vi "Loop_Auto.vi"() -> ()   [LabVIEW 2016, in "TemplateAutonomous.lvlib"]
uses:
  TemplateAutonomous.lvlib
  ENUM_Auto_State.ctl
  ENUM_Auto_Action.ctl
  Globals/Global_STOP.vi
panel:
  out "Input DBL Data":dbl
  out "Output Bool Data":bool
  out "Output DBL Data":dbl
  out "OutputI INT Data":i32
  out "Cycle Time (S)":dbl format="%.3g"
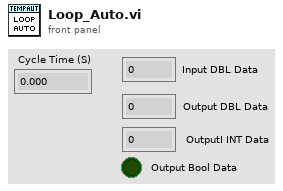
[diagram p1: front panel]
types:
  T1 = typedef "TemplateAutonomous.lvlib/ENUM_Auto_State.ctl" = enum16{"Startup", "Idle", "Auto Step 1", "Auto Step 2", "Shutdown"}
  T2 = typedef "TemplateAutonomous.lvlib/ENUM_Auto_Action.ctl" = enum16{"No Action", "Reset Time", "Reset All", "Action A", "Action B"}
  T3 = cluster{"State":T1, "Previous State":T1, "Current Time":timestamp, "Previous Time":timestamp, "Start Time":timestamp, "Target Time (ms)":u32, "Cycle Time(S)":dbl, "Auto Input DBL":dbl, "Auto Output DBL":dbl, "Auto OutputI INT":i32, "Auto Output Bool":bool}
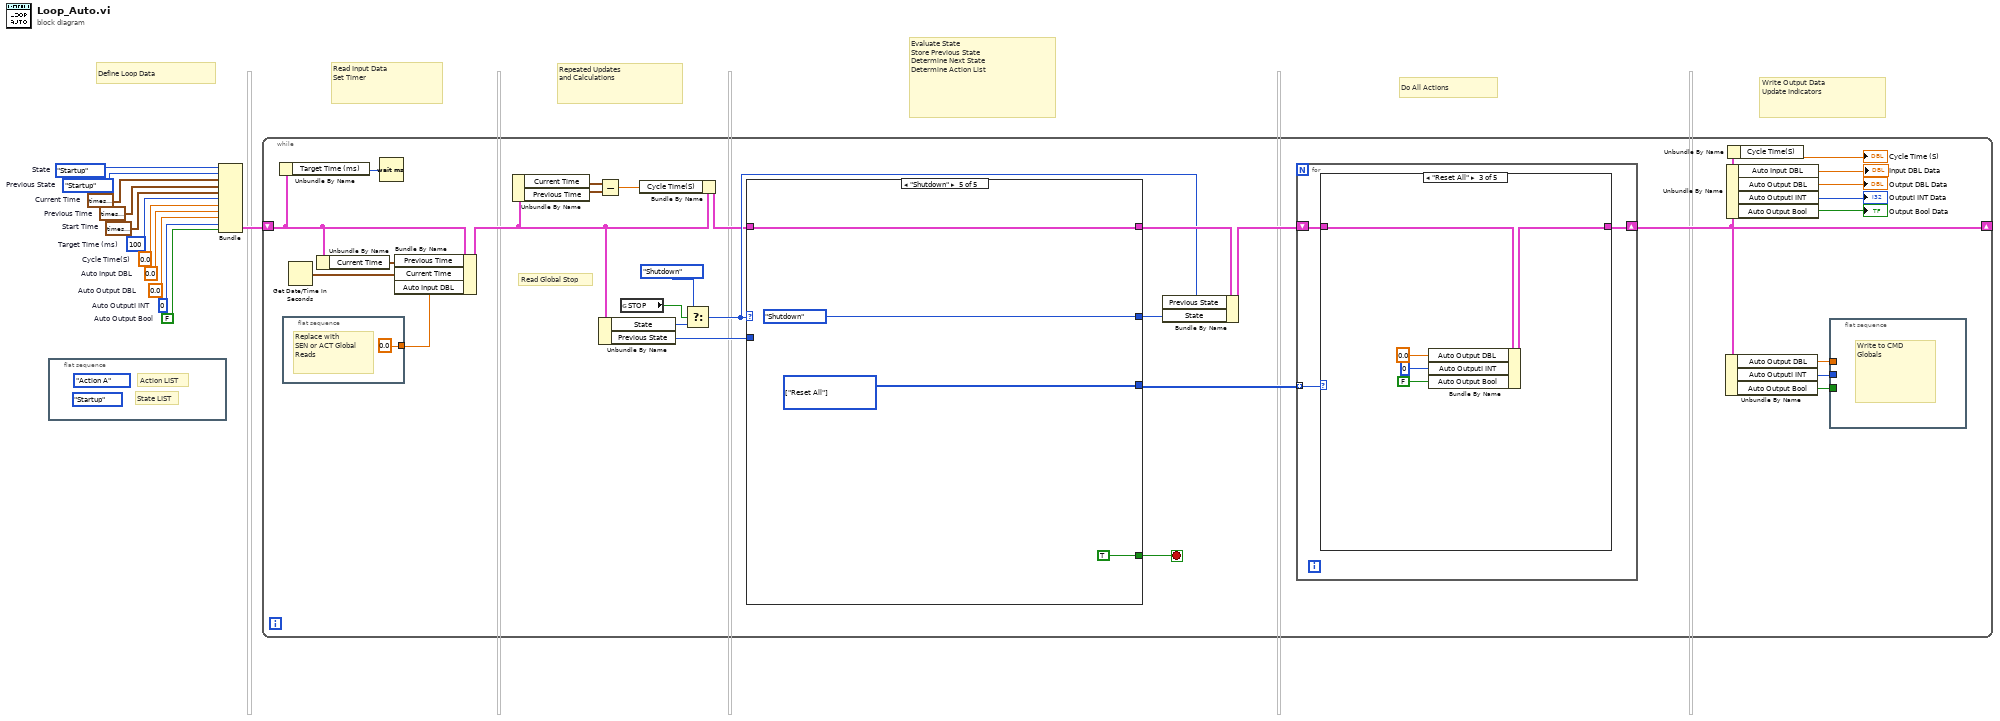
[diagram p0: block diagram]
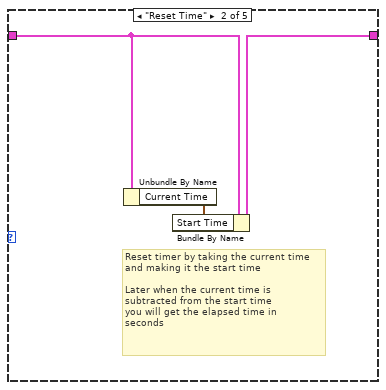
[diagram p3: hidden frame]
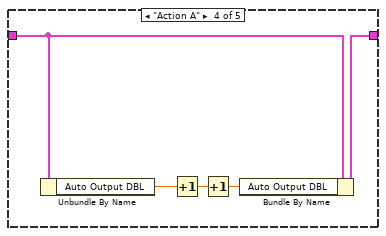
[diagram p4: hidden frame]
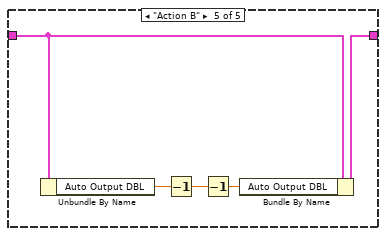
[diagram p5: hidden frame]
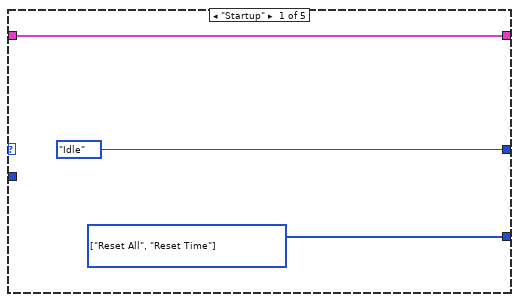
[diagram p6: hidden frame]
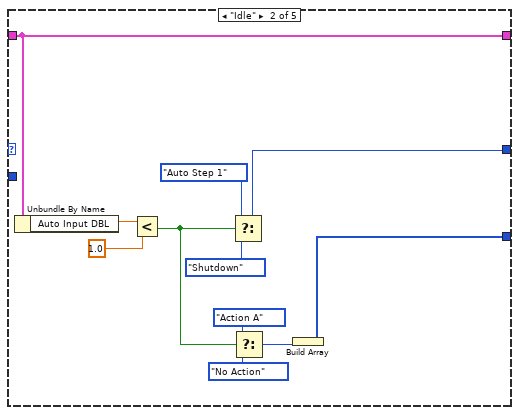
[diagram p7: hidden frame]
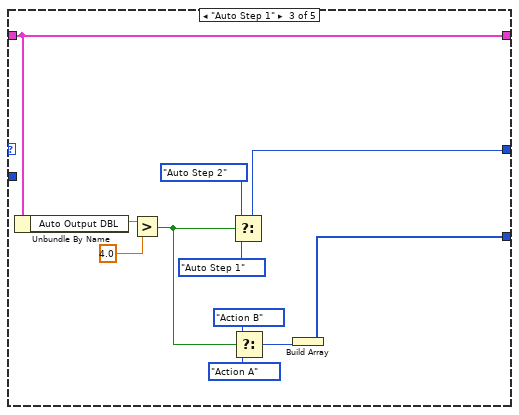
[diagram p8: hidden frame]
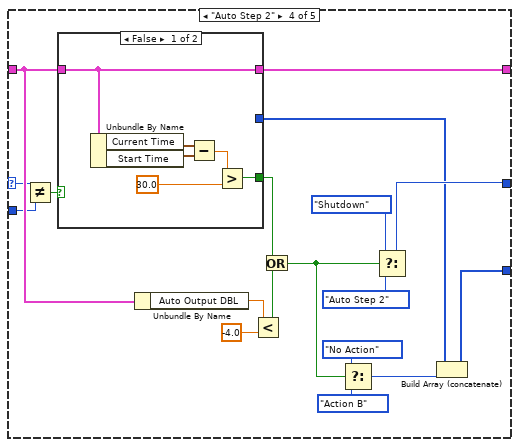
[diagram p9: hidden frame]
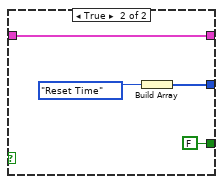
[diagram p10: hidden frame]
diagram:
  w1 = 0.0  # Cycle Time(S)
  w2 = ENUM_Auto_State."Startup"  # Previous State
  w3 = timestamp(0 s since 1904-01-01)  # Previous Time
  w4 = FALSE  # Auto Output Bool
  w5 = 0  # Auto OutputI INT
  w6 = u32 100  # Target Time (ms)
  w7 = 0.0  # Auto Output DBL
  w8 = 0.0  # Auto Input DBL
  w9 = timestamp(0 s since 1904-01-01)  # Start Time
  w10 = timestamp(0 s since 1904-01-01)  # Current Time
  w11 = ENUM_Auto_State."Startup"  # State
  # "Define Loop Data"
  # "Repeated Updates\nand Calculations"
  # "Read Input Data\nSet Timer"
  # "Evaluate State\nStore Previous State\nDetermine Next State\nDetermine Action List"
  # "Do All Actions"
  # "Write Output Data\nUpdate Indicators"
  n1 = flat-sequence {
    frame #0 {
      (unwired) ENUM_Auto_State."Startup" ("State")
      (unwired) ENUM_Auto_Action."Action A" ("Action")
      # "State LIST"
      # "Action LIST"
    }
  }
  n2 = Bundle("State"=w11, "Previous State"=w2, "Current Time"=w10, "Previous Time"=w3, "Start Time"=w9, "Target Time (ms)"=w6, "Cycle Time(S)"=w1, "Auto Input DBL"=w8, "Auto Output DBL"=w7, "Auto OutputI INT"=w5, "Auto Output Bool"=w4) -> (w12:T3)  [unwired: 1 in]
  n3 = while {
    shift-right: [w25] -> _
    shift-left: w12 -> [w31]
    stop <- w13 stop-if-true
    # "Read Global Stop"
    n4 = Unbundle By Name(w31) -> ("Target Time (ms)"=w34:u32)
    n5 = flat-sequence {
      tunnel: [0.0] -> w33
      frame #0 {
        # "Replace with \nSEN or ACT Global \nReads"
      }
    }
    n6 = Get Date/Time In Seconds() -> (seconds since 1Jan1904=w41:timestamp)
    n7 = Unbundle By Name(w31) -> ("Current Time"=w32:timestamp)
    n8 = Wait (ms)(milliseconds to wait=w34) -> ()  [unwired: 1 out]
    n9 = Bundle By Name(cluster=w31, "Previous Time"=w32, "Current Time"=w41, "Auto Input DBL"=w33) -> (w21:T3)
    n10 = Unbundle By Name(w21) -> ("Current Time"=w22:timestamp, "Previous Time"=w23:timestamp)
    n11 = Subtract(x=w22, y=w23) -> (x-y=w19:dbl)
    n12 = Unbundle By Name(w21) -> ("State"=w35:T1, "Previous State"=w30:T1)
    n13 = global read "Global_STOP.vi" "STOP"() -> (w37:bool)
    n14 = Bundle By Name(cluster=w21, "Cycle Time(S)"=w19) -> (w20:T3)
    n15 = Select(t=ENUM_Auto_State."Shutdown" ("State"), s=w37, f=w35) -> (s? t:f=w26:T1)
    n16 = case shown="\"Shutdown\"" w26 {
      selector: w26 -> [_ _ _ w93 _]
      tunnel: w20 -> [w67 w78 w89 w95 w121]
      tunnel: [w67 w78 w89 w94 w121] -> w39
      tunnel: [ENUM_Auto_State."Idle" ("State") w77 w88 w107 ENUM_Auto_State."Shutdown" ("State")] -> w38
      tunnel: [w66 w70 w81 w100 w119] -> w18
      tunnel: w30 -> [_ _ _ w92 _]
      tunnel: [_ _ _ _ TRUE] -> w13
      frame "Startup" {
        w66 = T2[] [enum."Reset All", enum."Reset Time"] items=["No Action", "Reset Time", "Reset All", "Action A", "Action B"] ("Actions")
      }
      frame "Idle" {
        n17 = Unbundle By Name(w78) -> ("Auto Input DBL"=w69:dbl)
        n18 = Less?(x=w69, y=1.0) -> (x < y?=w72:bool)
        n19 = Select(t=ENUM_Auto_State."Auto Step 1" ("State"), s=w72, f=ENUM_Auto_State."Shutdown" ("State")) -> (s? t:f=w77:T1)
        n20 = Select(t=ENUM_Auto_Action."Action A" ("Action"), s=w72, f=ENUM_Auto_Action."No Action" ("Action")) -> (s? t:f=w71:T2)
        n21 = Build Array(w71) -> (w70:T2[])
      }
      frame "Auto Step 1" {
        n22 = Unbundle By Name(w89) -> ("Auto Output DBL"=w80:dbl)
        n23 = Greater?(x=w80, y=4.0) -> (0:w83:bool)
        n24 = Select(t=ENUM_Auto_State."Auto Step 2" ("State"), s=w83, f=ENUM_Auto_State."Auto Step 1" ("State")) -> (s? t:f=w88:T1)
        n25 = Select(t=ENUM_Auto_Action."Action B" ("Action"), s=w83, f=ENUM_Auto_Action."Action A" ("Action")) -> (s? t:f=w82:T2)
        n26 = Build Array(w82) -> (w81:T2[])
      }
      frame "Auto Step 2" {
        n27 = Not Equal?(x=w93, y=w92) -> (x != y?=w91:bool)
        n28 = case shown="False" w91 {
          tunnel: [w113 FALSE] -> w102
          tunnel: w95 -> [w108 w116]
          tunnel: [w108 w116] -> w94
          tunnel: [_ w114] -> w90
          frame False {
            n29 = Unbundle By Name(w108) -> ("Current Time"=w111:timestamp, "Start Time"=w110:timestamp)
            n30 = Subtract(x=w111, y=w110) -> (x-y=w109:dbl)
            n31 = Greater?(x=w109, y=30.0) -> (0:w113:bool)
          }
          frame True {
            n32 = Build Array(ENUM_Auto_Action."Reset Time" ("Action")) -> (w114:T2[])
          }
        }
        n33 = Unbundle By Name(w95) -> ("Auto Output DBL"=w98:dbl)
        n34 = Less?(x=w98, y=-4.0) -> (x < y?=w96:bool)
        n35 = Or(x=w102, y=w96) -> (x .or. y?=w99:bool)
        n36 = Select(t=ENUM_Auto_Action."No Action" ("Action"), s=w99, f=ENUM_Auto_Action."Action B" ("Action")) -> (s? t:f=w101:T2)
        n37 = Select(t=ENUM_Auto_State."Shutdown" ("State"), s=w99, f=ENUM_Auto_State."Auto Step 2" ("State")) -> (s? t:f=w107:T1)
        n38 = Build Array (concatenate)(w90, w101) -> (w100:T2[])
      }
      frame "Shutdown" {
        w119 = T2[] [enum."Reset All"] items=["No Action", "Reset Time", "Reset All", "Action A", "Action B"] ("Actions")
      }
    }
    n39 = Bundle By Name(cluster=w39, "Previous State"=w26, "State"=w38) -> (w40:T3)
    n40 = for {
      tunnel: w18 -> [w45] mode=indexing
      shift-right: [w44] -> w25
      shift-left: w40 -> [w43]
      n41 = case shown="\"Reset All\"" w45 {
        tunnel: w43 -> [w46 w49 w54 w58 w63]
        tunnel: [w46 w48 w53 w57 w62] -> w44
        frame "No Action" {
        }
        frame "Reset Time" {
          # "Reset timer by taking the current time\nand making it the start time\n\nLater when the current time is \nsubtracted from the start time\nyou will get the elapsed time in \nseconds"
          n42 = Unbundle By Name(w49) -> ("Current Time"=w47:timestamp)
          n43 = Bundle By Name(cluster=w49, "Start Time"=w47) -> (w48:T3)
        }
        frame "Reset All" {
          n44 = Bundle By Name(cluster=w54, "Auto Output DBL"=0.0 ("FG Write Value"), "Auto OutputI INT"=0 ("OutputI INT"), "Auto Output Bool"=FALSE ("Output Bool")) -> (w53:T3)
        }
        frame "Action A" {
          n45 = Unbundle By Name(w58) -> ("Auto Output DBL"=w59:dbl)
          n46 = Increment(x=w59) -> (x+1=w55:dbl)
          n47 = Increment(x=w55) -> (x+1=w56:dbl)
          n48 = Bundle By Name(cluster=w58, "Auto Output DBL"=w56) -> (w57:T3)
        }
        frame "Action B" {
          n49 = Unbundle By Name(w63) -> ("Auto Output DBL"=w64:dbl)
          n50 = Decrement(x=w64) -> (x-1=w60:dbl)
          n51 = Decrement(x=w60) -> (x-1=w61:dbl)
          n52 = Bundle By Name(cluster=w63, "Auto Output DBL"=w61) -> (w62:T3)
        }
      }
    }
    n53 = Unbundle By Name(w25) -> ("Auto Output DBL"=w16:dbl, "Auto OutputI INT"=w15:i32, "Auto Output Bool"=w14:bool)
    n54 = Unbundle By Name(w25) -> ("Auto Input DBL"=→"Input DBL Data":dbl, "Auto Output DBL"=→"Output DBL Data":dbl, "Auto OutputI INT"=→"OutputI INT Data":i32, "Auto Output Bool"=→"Output Bool Data":bool)
    n55 = Unbundle By Name(w25) -> ("Cycle Time(S)"=→"Cycle Time (S)":dbl)
    n56 = flat-sequence {
      tunnel: w16 -> [_]
      tunnel: w15 -> [_]
      tunnel: w14 -> [_]
      frame #0 {
        # "Write to CMD\nGlobals"
      }
    }
  }
